vi "ReportHead_A131258.vi"(8 "error in (no error)":errorcluster caption="错误输入（无错误）", 11 "产品状态":string) -> (0 "error out":errorcluster caption="错误输出", 3 "report out":refnum<class "NI_report.lvclass"> caption="报表输出")   [LabVIEW 2020]
uses:
  <vilib>/Utility/NIReport.llb/NI_report.lvclass
  <vilib>/addons/_office/_exclsub.llb/font.ctl
  <vilib>/Utility/NIReport.llb/Report Type.ctl
  Database/Global1.vi
  Global_Variable/Global.vi
  <vilib>/addons/_office/NI_ReportGenerationToolkit.lvlib
  <vilib>/Utility/NIReport.llb/NI_ReportGenerationCore.lvlib
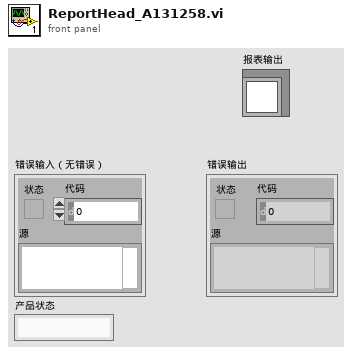
[diagram p1: front panel]
types:
  T1 = typedef "NI_ReportGenerationCore.lvlib/Report Type.ctl" = enum16{"HTML", "Word", "Excel"}
  T2 = cluster{"操作者编号":string, "操作者姓名":string, "操作者权限":string, "联机状态":string, "产品型号":string, "产品状态":string}
  T3 = cluster{"top":dbl, "left":dbl, "right":dbl, "bottom":dbl}
  T4 = cluster{"Charset (-1)":i16, "Weight (-1)":i16, "Name":string, "Size":string}
  T5 = cluster{"Italic":enum16{"Italic Unchanged", "Italic On", "Italic Off"}, "Strike Through":enum16{"Strike Through Unchanged", "Strike Through On", "Strike Through Off"}, "Underline":enum16{"Underline Unchanged", "Underline On", "Underline Off"}, "Bold":enum16{"Bold Unchanged", "Bold On", "Bold Off"}}
  T6 = typedef "NI_ReportGenerationToolkit.lvlib/font.ctl" = cluster{"font name":string, "font size":dbl, "bold":u16, "italic":u16, "underline":u16, "strike through":u16, "font color":u32}
  T7 = enum16{"maximized", "minimized", "normal", "no change"}
  T8 = cluster{"用户编号":string, "用户名":string, "用户密码(密文)":string, "用户权限":string}
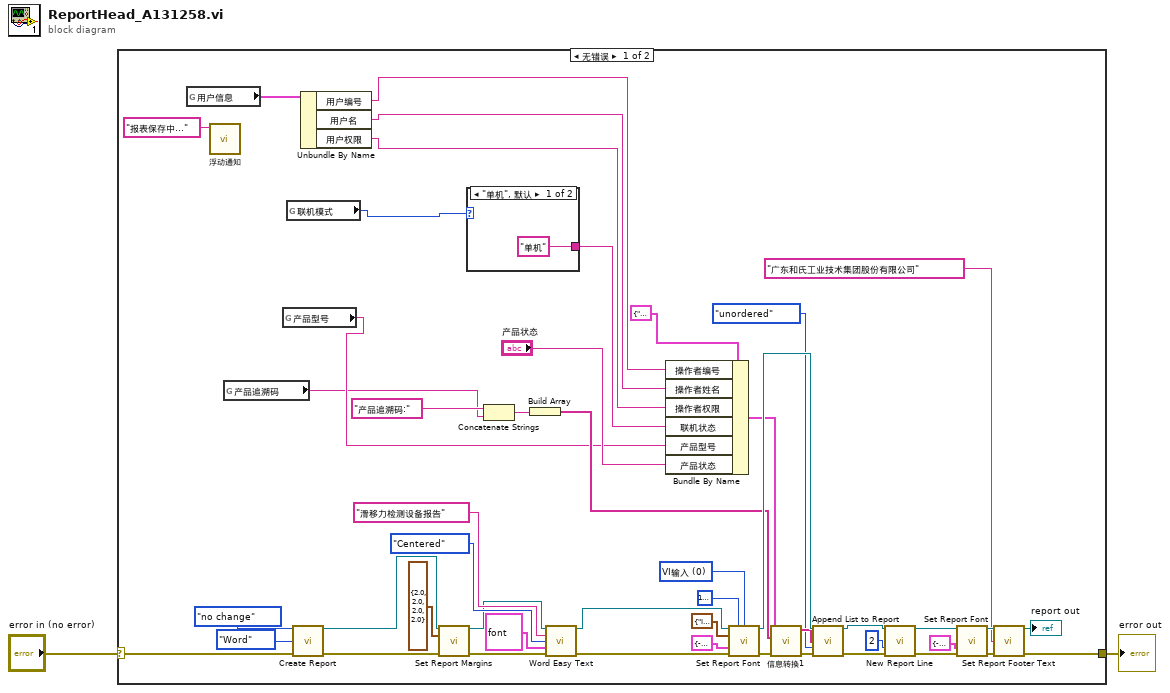
[diagram p0: block diagram]
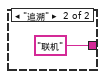
[diagram p2: hidden frame]
diagram:
  n1 = case shown="无错误" "error in (no error)" {
    selector: "error in (no error)" -> [w13 w53]
    tunnel: [w24 w53] -> w1
    frame No Error {
      w45 = u16 0 items=["VI输入", "字体对话框"] ("font settings source")
      n2 = global read "Global1.vi" "用户信息"() -> (w9:T8)
      n3 = call "浮动通知.vi"("通知内容"="报表保存中...") -> ()  [unwired: 11 in]
      n4 = global read "Global.vi" "产品追溯码"() -> (w4:string)
      n5 = global read "Global1.vi" "产品型号"() -> (w5:string)
      n6 = global read "Global1.vi" "联机模式"() -> (w10:enum16{"单机", "追溯"})
      n7 = call <vilib>:"Create Report.vi"("window state (normal)"=T7."no change", "report type"=Report_Type."Word", "error in (no error)"=w13) -> ("report out"=w11:refnum<class "NI_report.lvclass">, "error out"=w14:errorcluster)  [unwired: 11 in]
      n8 = Unbundle By Name(w9) -> ("用户编号"=w8:string, "用户名"=w7:string, "用户权限"=w6:string)
      n9 = call-dynamic "Set Report Margins.vi"("report in"=w11, "margins (1.00)"=T3 {"top"=2.0, "left"=2.0, "right"=2.0, "bottom"=2.0}, "error in (no error)"=w14) -> ("report out"=w38:refnum<class "NI_report.lvclass">, "error out"=w37:errorcluster)  [unwired: 10 in, 1 out]
      n10 = case shown="\"单机\", 默认" w10 {
        tunnel: ["单机" "联机"] -> w22
        frame "单机", Default {
        }
        frame "追溯" {
        }
      }
      n11 = Concatenate Strings("产品追溯码:", w4) -> (w18:string)
      n12 = Build Array(w18) -> (w17:string[])
      n13 = call <vilib>:"Word Easy Text.vi"("report in"=w38, "text"="滑移力检测设备报告", "alignment (left)"=enum16{"Left", "Centered", "Right", "Justify"}."Centered", "font"=T6 {"font name"="楷体", "font size"=26.0, "bold"=1, "italic"=2, "underline"=2, "strike through"=2, "font color"=16777228}, "error in (no error)"=w37) -> ("report out"=w47:refnum<class "NI_report.lvclass">, "error out"=w46:errorcluster)  [unwired: 8 in, 1 out]
      n14 = Bundle By Name(cluster=T2 {"操作者编号"="001", "操作者姓名"="Administrator", "操作者权限"="系统管理员", "联机状态"="单机", "产品型号"="SL7202", "产品状态"=""} ("测试信息"), "操作者编号"=w8, "操作者姓名"=w7, "操作者权限"=w6, "联机状态"=w22, "产品型号"=w5, "产品状态"="产品状态") -> (w20:T2)
      n15 = call-dynamic "Set Report Font.vi"("report in"=w47, "text color (unchanged)"=u32 16777224, "font settings source (VI Inputs)"=w45, "text options"=T5 {"Italic"=enum."Italic Off", "Strike Through"=enum."Strike Through Unchanged", "Underline"=enum."Underline Off", "Bold"=enum."Bold Off"}, "font settings"=T4 {"Charset (-1)"=-1, "Weight (-1)"=-1, "Name"="微软雅黑 Light", "Size"="12 "}, "error in (no error)"=w46) -> ("report out"=w35:refnum<class "NI_report.lvclass">, "error out"=w27:errorcluster)  [unwired: 7 in, 1 out]
      n16 = call "信息转换1.vi"("错误输入（无错误）"=w27, "追溯码"=w17, "测试信息"=w20) -> ("错误输出"=w26:errorcluster, "信息输出"=w28:string[])  [unwired: 7 in]
      n17 = call-dynamic "Append List to Report.vi"("report in"=w35, "list elements"=w28, "list type (ordered)"=enum16{"unordered", "ordered"}."unordered", "error in (no error)"=w26) -> ("report out"=w30:refnum<class "NI_report.lvclass">, "error out"=w29:errorcluster)  [unwired: 8 in, 2 out]
      n18 = call-dynamic "New Report Line.vi"("report in"=w30, "number of lines (1)"=2, "error in (no error)"=w29) -> ("report out"=w33:refnum<class "NI_report.lvclass">, "error out"=w34:errorcluster)  [unwired: 11 in]
      n19 = call-dynamic "Set Report Font.vi"("report in"=w33, "font settings"=T4 {"Charset (-1)"=-1, "Weight (-1)"=-1, "Name"="楷体", "Size"="9 "}, "error in (no error)"=w34) -> ("report out"=w42:refnum<class "NI_report.lvclass">, "error out"=w41:errorcluster)  [unwired: 10 in, 1 out]
      n20 = call-dynamic "Set Report Footer Text.vi"("report in"=w42, "center footer text"="广东和氏工业技术集团股份有限公司", "error in (no error)"=w41) -> ("report out"=→"report out":refnum<class "NI_report.lvclass">, "error out"=w24:errorcluster)  [unwired: 11 in]
    }
    frame Error {
    }
  }
  "error out" <- w1
